vi "Init LaunchPad.vi"(8 "error in":errorcluster, 10 "Baud Rate (9600)":u32=9600, 11 "VISA resource":refnum<visa-resource-name>) -> (0 "error out":errorcluster, 3 "VISA resource name out":refnum<visa-resource-name>)   [LabVIEW 2012]
doc: "Initializes a connection to an Arduino running the LabVIEW Interface for Arduino sketch.\n\nNote: The baud rate specified must match the baud rate defined by DEFAULTBAUDRATE in the Arduino firmware.\n\nNote: The Bytes Per Packet input must match the COMMANDLENGTH specified in the Arduino firmware."
uses:
  <vilib>/Instr/_visa.llb/VISA Configure Serial Port (Instr).vi
panel:
  in  "MaxNumTimeouts(20)":u32=20
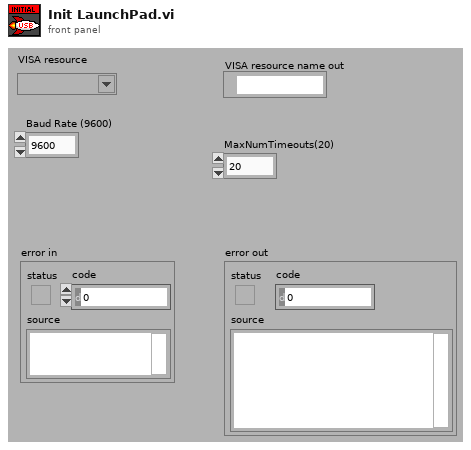
[diagram p1: front panel]
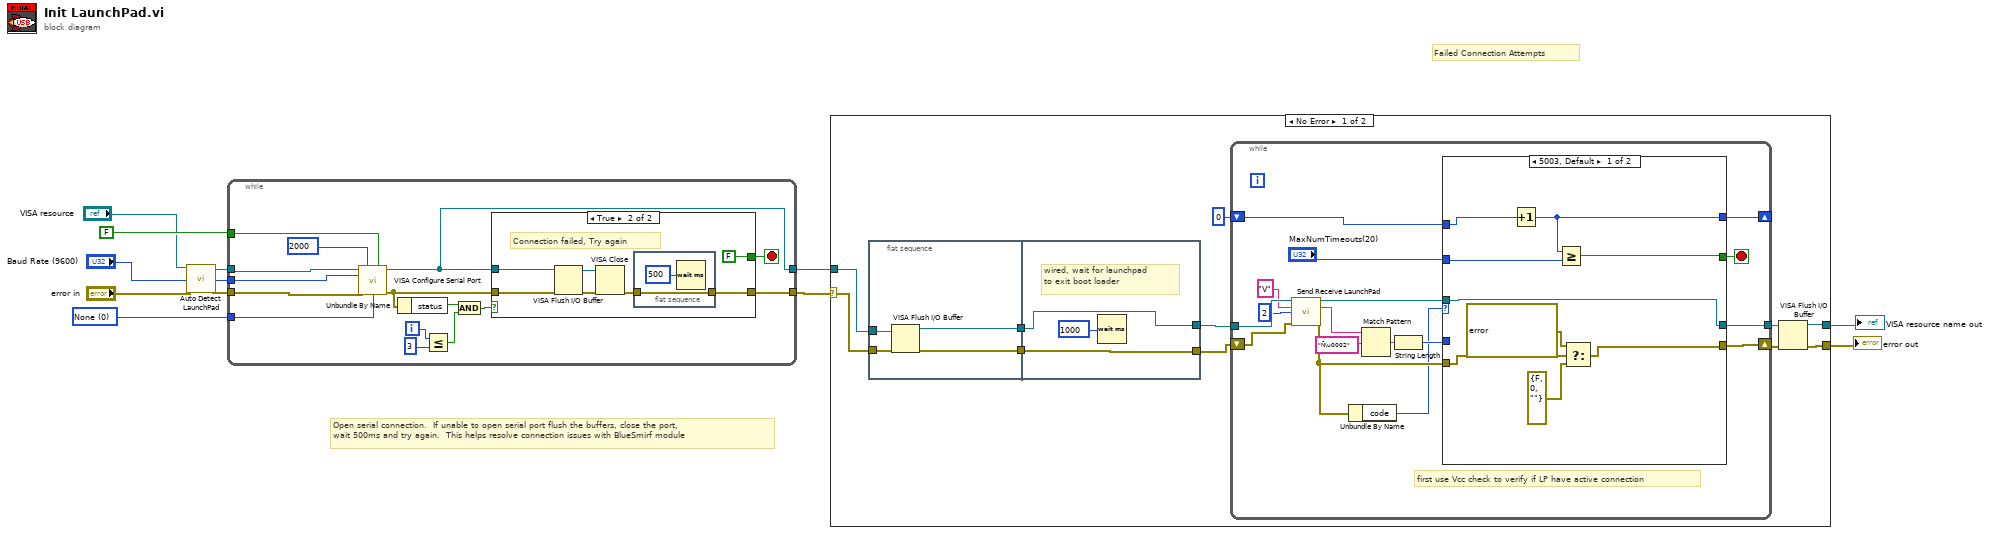
[diagram p0: block diagram]
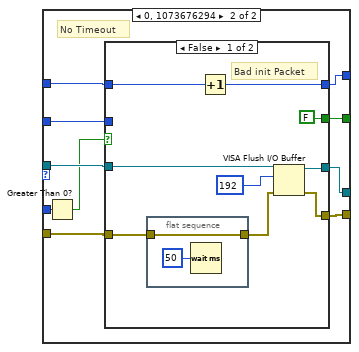
[diagram p2: hidden frame]
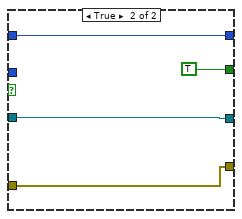
[diagram p3: hidden frame]
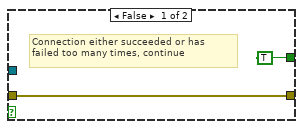
[diagram p5: hidden frame]
diagram:
  w11 = u16 0 items=["None", "XON/XOFF", "RTS/CTS", "XON/XOFF & RTS/CTS", "DTR/DSR", "XON/XOFF & DTR/DSR"] ("flow control (0:none)")
  # "Failed Connection Attempts"
  # "Open serial connection.  If unable to open serial port flush the buffers, close the port,\nwait 500ms and try again.  This helps resolve connection issues with BlueSmirf module"
  n1 = call "Auto Detect LaunchPad.vi"("Visa Resource"="VISA resource", "error in (no error)"="error in") -> ("VISA resource"=w8:refnum<visa-resource-name>, "error out"=w5:errorcluster)  [unwired: 12 in]
  n2 = while {
    tunnel: w11 -> [w26]
    tunnel: FALSE ("Enable Termination\nChar (T)") -> [w25]
    tunnel: "Baud Rate (9600)" -> [w24]
    tunnel: w8 -> [w13]
    tunnel: [w17] -> w1
    tunnel: [w15] -> w3
    tunnel: w5 -> [w12]
    i -> [w22]
    stop <- w16 stop-if-true
    n3 = call-poly "VISA Configure Serial Port"("VISA resource name"=w13, "timeout (10sec)"=u32 2000, "Enable Termination\nChar (T)"=w25, "baud rate (9600)"=w24, "error in (no error)"=w12, "flow control (0:none)"=w26) -> ("VISA resource name out"=w15:refnum<visa-resource-name>, "error out"=w18:errorcluster)  [unwired: 8 in]
    n4 = Unbundle By Name(w18) -> ("status"=w20:bool)
    n5 = Less Or Equal?(x=w22, y=3) -> (x <= y?=w21:bool)
    n6 = And(x=w20, y=w21) -> (x .and. y?=w19:bool)
    n7 = case shown="True" w19 {
      tunnel: w18 -> [w28 w31]
      tunnel: [w28 w30] -> w17
      tunnel: [TRUE FALSE] -> w16
      tunnel: w15 -> [_ w34]
      frame False {
        # "Connection either succeeded or has \nfailed too many times, continue"
      }
      frame True {
        # "Connection failed, Try again"
        n8 = VISA Flush I/O Buffer(VISA resource name=w34, error in (no error)=w31) -> (VISA resource name out=w33:refnum<visa-resource-name>, error out=w32:errorcluster)  [unwired: 1 in]
        n9 = VISA Close(VISA resource name=w33, error in (no error)=w32) -> (error out=w29:errorcluster)
        n10 = flat-sequence {
          tunnel: [w36] -> w30
          tunnel: w29 -> [w36]
          frame #0 {
            n11 = Wait (ms)(milliseconds to wait=u32 500) -> ()  [unwired: 1 out]
          }
        }
      }
    }
  }
  n12 = case shown="No Error" w1 {
    selector: w1 -> [w42 w107]
    tunnel: [w40 w107] -> w4
    tunnel: w3 -> [w47 w108]
    tunnel: [w38 w108] -> w2
    frame No Error {
      n13 = flat-sequence {
        tunnel: [w102] -> w48
        tunnel: w42 -> [w103]
        tunnel: w47 -> [w101]
        tunnel: [w100] -> w46
        tunnel: [w106] -> w44
        tunnel: w48 -> [w106]
        tunnel: w46 -> [w104]
        tunnel: [w104] -> w43
        frame #0 {
          n14 = VISA Flush I/O Buffer(VISA resource name=w101, error in (no error)=w103) -> (VISA resource name out=w100:refnum<visa-resource-name>, error out=w102:errorcluster)  [unwired: 1 in]
        }
        frame #1 {
          # "wired, wait for launchpad \nto exit boot loader"
          n15 = Wait (ms)(milliseconds to wait=u32 1000) -> ()  [unwired: 1 out]
        }
      }
      n16 = while {
        shift-right: [w56] -> _
        shift-left: 0 -> [w65]
        shift-right: [w51] -> w41
        shift-left: w44 -> [w63]
        tunnel: w43 -> [w64]
        tunnel: [w52] -> w39
        stop <- w55 stop-if-true
        # "first use Vcc check to verify if LP have active connection"
        n17 = call "Send Receive LaunchPad.vi"("VISA resource"=w64, "write buffer"="V", "Bytes To Read (0)"=u8 2, "error in"=w63) -> ("VISA resource 2"=w53:refnum<visa-resource-name>, "Read Buffer"=w60:string, "error out"=w50:errorcluster)  [unwired: 9 in]
        n18 = Unbundle By Name(w50) -> ("code"=w49:i32)
        n19 = Match Pattern(string=w60, regular expression="Ñ\u0002") -> (match substring=w59:string)  [unwired: 1 in, 3 out]
        n20 = String Length(string=w59) -> (length=w58:i32)
        n21 = case shown="5003, Default" w49 {
          tunnel: w65 -> [w74 w84]
          tunnel: w58 -> [_ w83]
          tunnel: [w71 w82] -> w56
          tunnel: [w72 w81] -> w55
          tunnel: "MaxNumTimeouts(20)" -> [w73 w80]
          tunnel: w53 -> [w66 w79]
          tunnel: [w66 w78] -> w52
          tunnel: [w67 w77] -> w51
          tunnel: w50 -> [w70 w76]
          frame 5003, Default {
            n22 = Increment(x=w74) -> (x+1=w71:i32)
            n23 = Greater Or Equal?(x=w71, y=w73) -> (x >= y?=w72:bool)
            n24 = Select(t=errorcluster {"status"=TRUE, "code"=5002, "source"="Init.vi.  Unable to establish connection with Arduino.  Please ensure that you have selected the correct COM port and that you have flashed the Arduino with the correct firmware."} ("error out"), s=w70, f=errorcluster {"status"=FALSE, "code"=0, "source"=""}) -> (s? t:f=w67:errorcluster)
          }
          frame 0, 1073676294 {
            # "No Timeout"
            n25 = Greater Than 0?(x=w83) -> (x > 0?=w75:bool)
            n26 = case shown="False" w75 {
              tunnel: w84 -> [w92 w99]
              tunnel: w80 -> [_ _]
              tunnel: [w91 w99] -> w82
              tunnel: [FALSE TRUE] -> w81
              tunnel: w79 -> [w89 w97]
              tunnel: [w88 w97] -> w78
              tunnel: w76 -> [w86 w96]
              tunnel: [w85 w96] -> w77
              frame False {
                # "Bad init Packet"
                n27 = flat-sequence {
                  tunnel: w86 -> [w94]
                  tunnel: [w94] -> w90
                  frame #0 {
                    n28 = Wait (ms)(milliseconds to wait=u32 50) -> ()  [unwired: 1 out]
                  }
                }
                n29 = Increment(x=w92) -> (x+1=w91:i32)
                n30 = VISA Flush I/O Buffer(VISA resource name=w89, mask (16)=u16 192, error in (no error)=w90) -> (VISA resource name out=w88:refnum<visa-resource-name>, error out=w85:errorcluster)
              }
              frame True {
              }
            }
          }
        }
      }
      n31 = VISA Flush I/O Buffer(VISA resource name=w39, error in (no error)=w41) -> (VISA resource name out=w38:refnum<visa-resource-name>, error out=w40:errorcluster)  [unwired: 1 in]
    }
    frame Error {
    }
  }
  "VISA resource name out" <- w2
  "error out" <- w4
